vi "Get w4lvgrpc_Msg_ToServer_5.vi"(8 "error in (no error)":errorcluster, 11 "gRPCid":T1) -> (0 "error out":errorcluster, 2 "package_templatemessage":T2, 3 "gRPCid out":T1)   [LabVIEW 2019, in "Generated_server.lvlib"]
uses:
  Generated_server.lvlib
  2ed25e12-861d-4677-8ead-ace2906b2041.vi
  w4lvgrpc_Msg_ToServer_5.ctl
  w4lvgrpc_Msg_ToServer_5_Flat.ctl
  <vilib>/gRPC/LabVIEW gRPC Library/Shared/grpcId.ctl
  <vilib>/gRPC/LabVIEW gRPC Library/grpc-lvsupport-release.lvlib
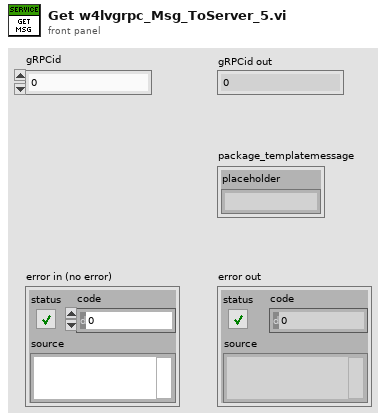
[diagram p1: front panel]
types:
  T1 = typedef "grpc-lvsupport-release.lvlib/grpcId.ctl" = u64
  T2 = typedef "Generated_server.lvlib/w4lvgrpc_Msg_ToServer_5.ctl" = cluster{"placeholder":string}
  T3 = typedef "Generated_server.lvlib/w4lvgrpc_Msg_ToServer_5_Flat.ctl" = cluster{"placeholder":string}
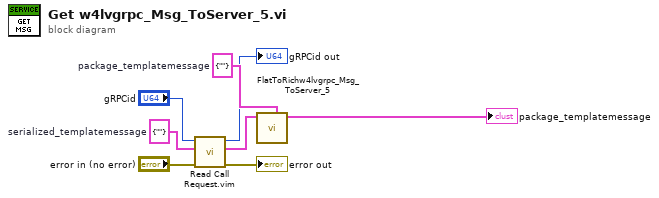
[diagram p0: block diagram]
diagram:
  w6 = T3 {"placeholder"=""}  # serialized_templatemessage
  w5 = T2 {"placeholder"=""}  # package_templatemessage
  n1 = call "Read Call Request.vim"("error in"="error in (no error)", "Request Type"=w6, "gRPCid in"="gRPCid") -> ("error out"=→"error out":errorcluster, "Request Data"=w4:T3, "gRPCid out"=→"gRPCid out":T1)  [unwired: 6 in]
  n2 = call "FlatToRichw4lvgrpc_Msg_ToServer_5.vi"("OutputClusterType"=w5, "InputCluster"=w4) -> ("OutputCluster"=→"package_templatemessage":T2)  [unwired: 9 in]
